vi "FlexRay_Demo_Template.vi"() -> ()   [LabVIEW 2014]
uses:
  TSMaster_API/FlexRay_Function/Typedef/TLibFLexRay.ctl
panel:
  out "FR_Buffer":T1[](array[typedef])
  # "使用方法：\n1.创建TSMaster 工程，使能两个通道进行桥接，并配置FlexRay数据库以及调度表\n2.保存TSMater 工程\n3.此demo 导入上述工程路径并进行创建APP\n4.运行此demo 发送报文并接收"
  # "usage method:\n1. Create TSMaster project to enable bridging of two channels and configure FlexRay database and scheduling table\n2. Save TSMater project\n3. Import the above project path into this demo and create an APP.\n4. Send and receive messages in this demo"
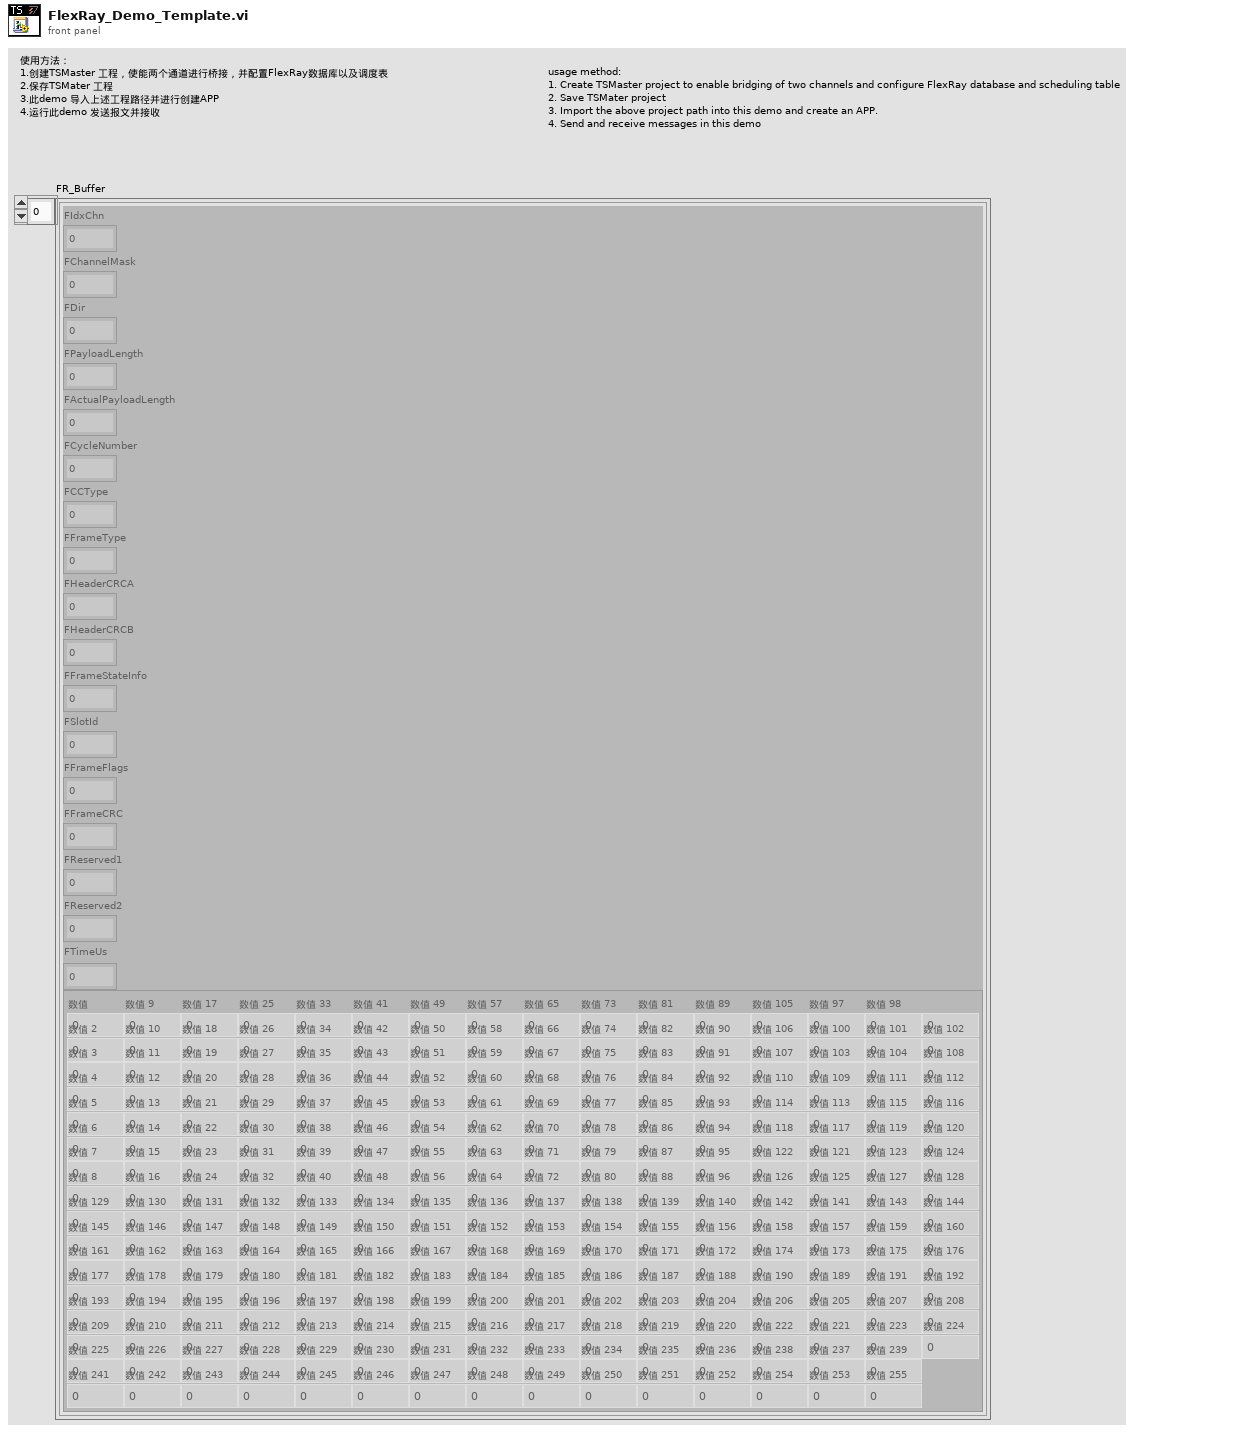
[diagram p1: front panel]
types:
  T1 = typedef "TLibFLexRay.ctl" = cluster{"FIdxChn":u8, "FChannelMask":u8, "FDir":u8, "FPayloadLength":u8, "FActualPayloadLength":u8, "FCycleNumber":u8, "FCCType":u8, "FFrameType":u8, "FHeaderCRCA":u16, "FHeaderCRCB":u16, "FFrameStateInfo":u16, "FSlotId":u16, "FFrameFlags":u32, "FFrameCRC":u32, "FReserved1":u64, "FReserved2":u64, "FTimeUs":u64, "FData":cluster{"数值":u8, "数值 9":u8, "数值 17":u8, "数值 25":u8, "数值 33":u8, "数值 41":u8, "数值 49":u8, "数值 57":u8, "数值 65":u8, "数值 73":u8, "数值 81":u8, "数值 89":u8, "数值 97":u8, "数值 105":u8, "数值 98":u8, "数值 99":u8, "数值 2":u8, "数值 10":u8, "数值 18":u8, "数值 26":u8, "数值 34":u8, "数值 42":u8, "数值 50":u8, "数值 58":u8, "数值 66":u8, "数值 74":u8, "数值 82":u8, "数值 90":u8, "数值 100":u8, "数值 106":u8, "数值 101":u8, "数值 102":u8, "数值 3":u8, "数值 11":u8, "数值 19":u8, "数值 27":u8, "数值 35":u8, "数值 43":u8, "数值 51":u8, "数值 59":u8, "数值 67":u8, "数值 75":u8, "数值 83":u8, "数值 91":u8, "数值 103":u8, "数值 107":u8, "数值 104":u8, "数值 108":u8, "数值 4":u8, "数值 12":u8, "数值 20":u8, "数值 28":u8, "数值 36":u8, "数值 44":u8, "数值 52":u8, "数值 60":u8, "数值 68":u8, "数值 76":u8, "数值 84":u8, "数值 92":u8, "数值 109":u8, "数值 110":u8, "数值 111":u8, "数值 112":u8, "数值 5":u8, "数值 13":u8, "数值 21":u8, "数值 29":u8, "数值 37":u8, "数值 45":u8, "数值 53":u8, "数值 61":u8, "数值 69":u8, "数值 77":u8, "数值 85":u8, "数值 93":u8, "数值 113":u8, "数值 114":u8, "数值 115":u8, "数值 116":u8, "数值 6":u8, "数值 14":u8, "数值 22":u8, "数值 30":u8, "数值 38":u8, "数值 46":u8, "数值 54":u8, "数值 62":u8, "数值 70":u8, "数值 78":u8, "数值 86":u8, "数值 94":u8, "数值 117":u8, "数值 118":u8, "数值 119":u8, "数值 120":u8, "数值 7":u8, "数值 15":u8, "数值 23":u8, "数值 31":u8, "数值 39":u8, "数值 47":u8, "数值 55":u8, "数值 63":u8, "数值 71":u8, "数值 79":u8, "数值 87":u8, "数值 95":u8, "数值 121":u8, "数值 122":u8, "数值 123":u8, "数值 124":u8, "数值 8":u8, "数值 16":u8, "数值 24":u8, "数值 32":u8, "数值 40":u8, "数值 48":u8, "数值 56":u8, "数值 64":u8, "数值 72":u8, "数值 80":u8, "数值 88":u8, "数值 96":u8, "数值 125":u8, "数值 126":u8, "数值 127":u8, "数值 128":u8, "数值 129":u8, "数值 130":u8, "数值 131":u8, "数值 132":u8, "数值 133":u8, "数值 134":u8, "数值 135":u8, "数值 136":u8, "数值 137":u8, "数值 138":u8, "数值 139":u8, "数值 140":u8, "数值 141":u8, "数值 142":u8, "数值 143":u8, "数值 144":u8, "数值 145":u8, "数值 146":u8, "数值 147":u8, "数值 148":u8, "数值 149":u8, "数值 150":u8, "数值 151":u8, "数值 152":u8, "数值 153":u8, "数值 154":u8, "数值 155":u8, "数值 156":u8, "数值 157":u8, "数值 158":u8, "数值 159":u8, "数值 160":u8, "数值 161":u8, "数值 162":u8, "数值 163":u8, "数值 164":u8, "数值 165":u8, "数值 166":u8, "数值 167":u8, "数值 168":u8, "数值 169":u8, "数值 170":u8, "数值 171":u8, "数值 172":u8, "数值 173":u8, "数值 174":u8, "数值 175":u8, "数值 176":u8, "数值 177":u8, "数值 178":u8, "数值 179":u8, "数值 180":u8, "数值 181":u8, "数值 182":u8, "数值 183":u8, "数值 184":u8, "数值 185":u8, "数值 186":u8, "数值 187":u8, "数值 188":u8, "数值 189":u8, "数值 190":u8, "数值 191":u8, "数值 192":u8, "数值 193":u8, "数值 194":u8, "数值 195":u8, "数值 196":u8, "数值 197":u8, "数值 198":u8, "数值 199":u8, "数值 200":u8, "数值 201":u8, "数值 202":u8, "数值 203":u8, "数值 204":u8, "数值 205":u8, "数值 206":u8, "数值 207":u8, "数值 208":u8, "数值 209":u8, "数值 210":u8, "数值 211":u8, "数值 212":u8, "数值 213":u8, "数值 214":u8, "数值 215":u8, "数值 216":u8, "数值 217":u8, "数值 218":u8, "数值 219":u8, "数值 220":u8, "数值 221":u8, "数值 222":u8, "数值 223":u8, "数值 224":u8, "数值 225":u8, "数值 226":u8, "数值 227":u8, "数值 228":u8, "数值 229":u8, "数值 230":u8, "数值 231":u8, "数值 232":u8, "数值 233":u8, "数值 234":u8, "数值 235":u8, "数值 236":u8, "数值 237":u8, "数值 238":u8, "数值 239":u8, "数值 241":u8, "数值 242":u8, "数值 243":u8, "数值 244":u8, "数值 245":u8, "数值 246":u8, "数值 247":u8, "数值 248":u8, "数值 249":u8, "数值 250":u8, "数值 251":u8, "数值 252":u8, "数值 253":u8, "数值 254":u8, "数值 255":u8}}
  T2 = cluster{"FIdxChn":u8, "FChannelMask":u8, "FActualPayloadLength":u8, "FCycleNumber":u8, "FSlotId":u16, "Send_Array":u8[]}
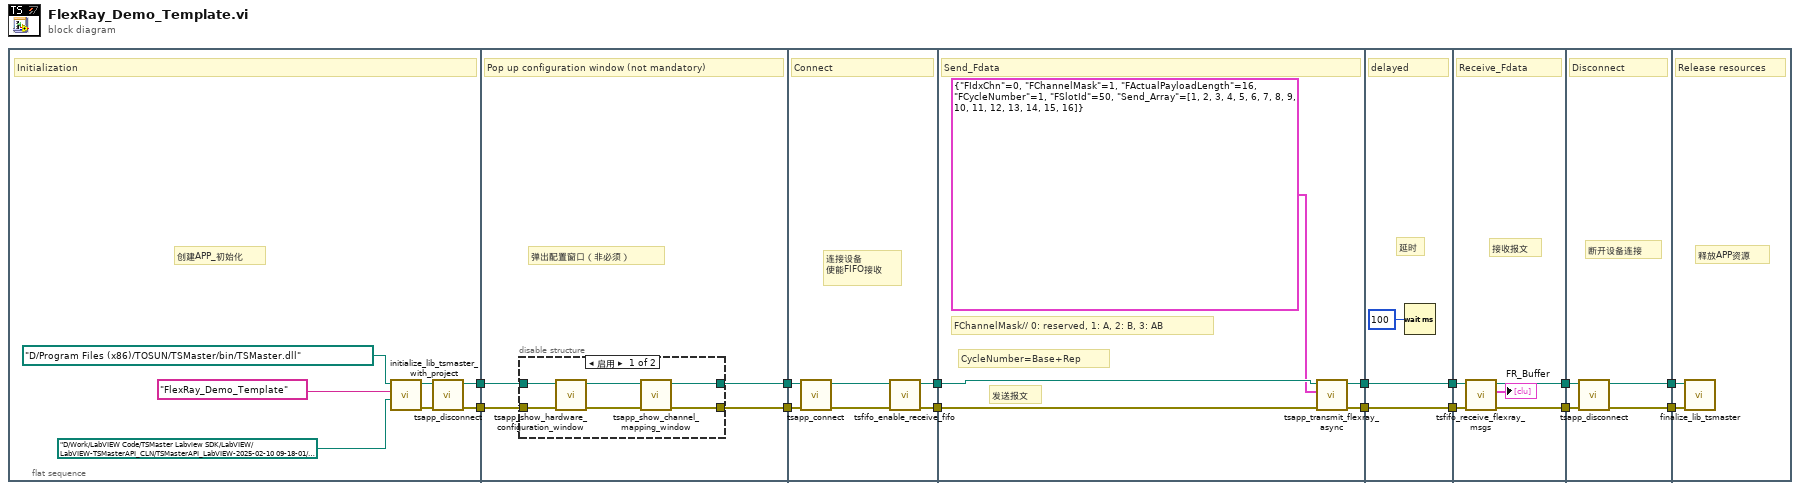
[diagram p0: block diagram]
diagram:
  n1 = flat-sequence {
    tunnel: [w21] -> w14
    tunnel: [w20] -> w13
    tunnel: w14 -> [w24]
    tunnel: w13 -> [w25]
    tunnel: [w23] -> w6
    tunnel: [w22] -> w5
    tunnel: [w37] -> w12
    tunnel: [w36] -> w11
    tunnel: w6 -> [w35]
    tunnel: w5 -> [w34]
    tunnel: w12 -> [w44]
    tunnel: w11 -> [w43]
    tunnel: [w42] -> w4
    tunnel: [w41] -> w2
    tunnel: w4 -> [w47]
    tunnel: [w47] -> w3
    tunnel: w2 -> [w46]
    tunnel: [w46] -> w1
    tunnel: [w50] -> w10
    tunnel: [w49] -> w9
    tunnel: w3 -> [w52]
    tunnel: w1 -> [w51]
    tunnel: w10 -> [w56]
    tunnel: w9 -> [w55]
    tunnel: [w54] -> w8
    tunnel: [w53] -> w7
    tunnel: w8 -> [w58]
    tunnel: w7 -> [w57]
    frame #0 {
      # "创建APP_初始化"
      # "Initialization"
      n2 = call "initialize_lib_tsmaster_with_project.vi"("projectfile"=path "D:/Work/LabVIEW Code/TSMaster Labview SDK/LabVIEW/LabVIEW-TSMasterAPI_CLN/TSMasterAPI_LabVIEW-2025-02-10 09-18-01/Demo/FlexRay/TSMaster_FlexRay", "AppName"="FlexRay_Demo_Template", "Path input"=path "D:/Program Files (x86)/TOSUN/TSMaster/bin/TSMaster.dll") -> ("error output"=w18:errorcluster, "Path output"=w19:path)  [unwired: 7 in]
      n3 = call "tsapp_disconnect.vi"("error in (no error)"=w18, "Path"=w19) -> ("error output"=w21:errorcluster, "Path output"=w20:path)  [unwired: 7 in, 1 out]
    }
    frame #1 {
      # "弹出配置窗口（非必须）"
      # "Pop up configuration window (not mandatory)"
      n4 = disable-structure shown="启用" {
        disable-tunnel: w25 -> [w31 w33]
        disable-tunnel: w24 -> [w30 w32]
        disable-tunnel: [w27 w33] -> w23
        disable-tunnel: [w26 w32] -> w22
        frame Enabled {
          n5 = call "tsapp_show_hardware_configuration_window.vi"("error in (no error)"=w30, "路径输入"=w31) -> ("error out"=w28:errorcluster, "路径输出"=w29:path)  [unwired: 7 in, 1 out]
          n6 = call "tsapp_show_channel_mapping_window.vi"("error in (no error)"=w28, "路径输入"=w29) -> ("error out"=w26:errorcluster, "路径输出"=w27:path)  [unwired: 7 in, 1 out]
        }
        frame Disabled {
        }
      }
    }
    frame #2 {
      # "连接设备\n使能FIFO接收"
      # "Connect"
      n7 = call "tsapp_connect.vi"("error in (no error)"=w34, "Path"=w35) -> ("error out"=w39:errorcluster, "Path output"=w38:path)  [unwired: 7 in, 1 out]
      n8 = call "tsfifo_enable_receive_fifo.vi"("error in (no error)"=w39, "Path"=w38) -> ("error out"=w36:errorcluster, "Path output"=w37:path)  [unwired: 8 in]
    }
    frame #3 {
      # "CycleNumber=Base+Rep"
      # "FChannelMask// 0: reserved, 1: A, 2: B, 3: AB"
      # "发送报文"
      # "Send_Fdata"
      n9 = call "tsapp_transmit_flexray_async.vi"("error in (no error)"=w43, "FR_Transmit"=T2 {"FIdxChn"=0, "FChannelMask"=1, "FActualPayloadLength"=16, "FCycleNumber"=1, "FSlotId"=50, "Send_Array"=[1, 2, 3, 4, 5, 6, 7, 8, 9, 10, 11, 12, 13, 14, 15, 16]}, "Path"=w44) -> ("error out"=w41:errorcluster, "Path output"=w42:path)  [unwired: 5 in, 1 out]
    }
    frame #4 {
      # "延时"
      # "delayed"
      n10 = Wait (ms)(milliseconds to wait=u32 100 ("等待时间（毫秒）")) -> ()  [unwired: 1 out]
    }
    frame #5 {
      # "接收报文"
      # "Receive_Fdata"
      n11 = call "tsfifo_receive_flexray_msgs.vi"("error in (no error)"=w51, "Path"=w52) -> ("error out"=w49:errorcluster, "FR_Buffer"=→"FR_Buffer":T1[], "Path output"=w50:path)  [unwired: 5 in, 1 out]
    }
    frame #6 {
      # "断开设备连接"
      # "Disconnect"
      n12 = call "tsapp_disconnect.vi"("error in (no error)"=w55, "Path"=w56) -> ("error output"=w54:errorcluster, "Path output"=w53:path)  [unwired: 7 in, 1 out]
    }
    frame #7 {
      # "释放APP资源"
      # "Release resources"
      n13 = call "finalize_lib_tsmaster.vi"("error in (no error)"=w58, "Path"=w57) -> ()  [unwired: 8 in, 2 out]
    }
  }
